vi "ReadConstantSpreadsheet.vi"(2 "error in":errorcluster, 3 "Constant":string="Drive Left Center", 4 "2020ConstantSpreadSheet":string[][](array[string])=[["Robot ID", "Motor ID", "Can Bus ID", "PWM Channel", "PDP Channel ID", "Breaker Needed", "Max. Allowed Current", "Solenoid Channel", "Analog Channel", "Digital I/O", "Notes", ""], ["981-2020", "Drive Right A", "11", "-1", "2", "40", "40", "-1", "-1", "-1", "", ""], ["981-2020", "Drive Right B", "12", "-1", "3", "40", "40", "-1", "-1", "-1", "", ""], ["981-2020", "Drive Left A", "13", "-1", "12", "40", "40", "-1", "-1", "-1", "", ""], ["981-2020", "Drive Left B", "14", "-1", "13", "40", "40", "-1", "-1", "-1", "", ""], ["981-2020", "Kicker", "15", "-1", "7", "20", "20", "-1", "-1", "-1", "", ""], ["981-2020", "Lift", "16", "-1", "6", "20", "20", "-1", "-1", "-1", "", ""], ["981-2020", "Shooter Left", "17", "-1", "1", "40", "40", "-1", "-1", "-1", "", ""], ["981-2020", "Shooter Right", "18", "-1", "0", "40", "40", "-1", "-1", "-1", "", ""], ["981-2020", "Pulley", "19", "-1", "5", "20", "20", "-1", "-1", "-1", "", ""], ["981-2020", "Intake", "20", "-1", "4", "20", "20", "-1", "-1", "-1", "", ""], ["981-2020", "Loader", "21", "-1", "11", "20", "20", "-1", "-1", "-1", "Changed name from spinner to the agreed name loader", ""], ["981-2020", "Winch", "22", "-1", "12", "20", "20", "-1", "-1", "-1", "", ""], ["981-2020", "Spare", "23", "-1", "8", "20", "20", "-1", "-1", "-1", "", ""], ["981S", "Drive Left Front", "0", "0", "0", "20", "20", "-1", "-1", "-1", "These are the IDs for the software sim of the 981 robot", ""], ["981S", "Drive Left Rear", "0", "1", "0", "20", "20", "-1", "-1", "-1", "", ""], ["981S", "Drive Right Front", "0", "0", "0", "20", "20", "-1", "-1", "-1", "", ""], ["981S", "Drive Right Rear", "0", "0", "0", "20", "20", "-1", "-1", "-1", "", ""], ["981S", "Gripper Left", "0", "0", "0", "20", "20", "-1", "-1", "-1", "", ""], ["981S", "Gripper Right", "0", "1", "0", "20", "20", "-1", "-1", "-1", "", ""], ["981S", "Winch Motor", "0", "0", "0", "20", "20", "-1", "-1", "-1", "", ""], ["981S", "Fork Lift Motor", "0", "1", "0", "20", "20", "-1", "-1", "-1", "", ""], ["981", "Drive Right A", "13", "-1", "13", "40", "28", "-1", "-1", "-1", "\"AKA", " drive right front\""], ["981", "Drive Right B", "14", "-1", "14", "40", "27", "-1", "-1", "-1", "\"AKA", " drive right rear\""], ["981", "Drive Left A", "11", "-1", "0", "40", "26", "-1", "-1", "-1", "\"AKA", " drive left front\""], ["981", "Drive Left B", "12", "-1", "1", "40", "25", "-1", "-1", "-1", "\"AKA", " drive left rear\""], ["981", "Winch", "15", "-1", "15", "40", "40", "-1", "-1", "-1", "", ""], ["981", "Arm", "17", "-1", "11", "30", "39", "-1", "-1", "-1", "", ""], ["981", "Arm Pot", "-1", "-1", "-1", "-1", "-1", "-1", "1", "-1", "Using Channel for Analog Input Channel", ""], ["981", "Arm Encoder", "-1", "-1", "-1", "-1", "-1", "-1", "-1", "0", "\"Digital IO for A", " add one for channel B\""], ["981", "Lights", "0", "0", "8", "20", "2", "-1", "-1", "-1", "\"20 amp is overkill", " but the minimum for the PDP\""], ["981", "Raspberry Pi", "0", "9", "10", "20", "3", "-1", "-1", "-1", "", ""], ["981", "Total PDP", "0", "0", "17", "120", "118", "-1", "-1", "-1", "", ""], ["981", "Extend Arm", "-1", "-1", "-1", "-1", "-1", "2", "-1", "-1", "", ""], ["981", "Retract Arm", "-1", "-1", "-1", "-1", "-1", "3", "-1", "-1", "", ""], ["981", "Shift Low", "-1", "-1", "-1", "-1", "-1", "6", "-1", "-1", "", ""], ["981", "Shift High", "-1", "-1", "-1", "-1", "-1", "7", "-1", "-1", "", ""], ["981", "Close Gripper", "-1", "-1", "-1", "-1", "-1", "0", "-1", "-1", "", ""], ["981", "Open Gripper", "-1", "-1", "-1", "-1", "-1", "1", "-1", "-1", "", ""], ["981", "Extend Hook", "-1", "-1", "-1", "-1", "-1", "4", "-1", "-1", "", ""], ["981", "Retract Hook", "-1", "-1", "-1", "-1", "-1", "5", "-1", "-1", "", ""], ["984", "Drive Left Front", "11", "-1", "0", "20", "20", "-1", "-1", "-1", "These are the IDS for the Rhino Robot practice robot", ""], ["984", "Drive Left Rear", "12", "-1", "1", "20", "20", "-1", "-1", "-1", "", ""], ["984", "Drive Left Center", "13", "-1", "2", "20", "20", "-1", "-1", "-1", "", ""], ["984", "Drive Right Front", "14", "-1", "12", "20", "20", "-1", "-1", "-1", "", ""], ["984", "Drive Right Rear", "15", "-1", "13", "20", "20", "-1", "-1", "-1", "", ""], ["984", "Drive Right Center", "16", "-1", "14", "20", "20", "-1", "-1", "-1", "", ""], ["984", "Gripper Left", "17", "-1", "8", "20", "20", "-1", "-1", "-1", "", ""], ["984", "Gripper Right", "18", "-1", "9", "20", "20", "-1", "-1", "-1", "", ""], ["984", "Winch", "19", "-1", "4", "20", "20", "-1", "-1", "-1", "", ""], ["984", "Fork Lift Motor", "20", "-1", "5", "20", "20", "-1", "-1", "-1", "", ""], ["985", "Drive Left Front", "11", "-1", "0", "20", "20", "-1", "-1", "-1", "These are the IDs for the AM drive practice robot", ""], ["985", "Drive Left Rear", "12", "-1", "1", "20", "20", "-1", "-1", "-1", "", ""], ["985", "Drive Right Front", "13", "-1", "2", "20", "20", "-1", "-1", "-1", "", ""], ["985", "Drive Right Rear", "14", "-1", "3", "20", "20", "-1", "-1", "-1", "", ""], ["985", "Gripper Left", "15", "-1", "10", "20", "20", "-1", "-1", "-1", "", ""], ["985", "Gripper Right", "16", "-1", "11", "20", "20", "-1", "-1", "-1", "", ""], ["985", "Winch Motor", "17", "-1", "14", "20", "20", "-1", "-1", "-1", "", ""], ["985", "Fork Lift Motor", "18", "-1", "5", "20", "20", "-1", "-1", "-1", "", ""], ["985SW", "Drive Right", "1", "-1", "1", "40", "20", "-1", "-1", "-1", "985 Summer Wheeled Robot right drive motor", ""], ["985SW", "Drive Left", "2", "-1", "1", "40", "20", "-1", "-1", "-1", "985 Summer Wheeled Robot left drive motor", ""], ["985SW", "Lift", "3", "-1", "1", "40", "20", "-1", "-1", "-1", "985 Lift Motor", ""]], 5 "Robot ID":string="984") -> (0 "error out":errorcluster, 1 "Constant Value":dbl)   [LabVIEW 2020]
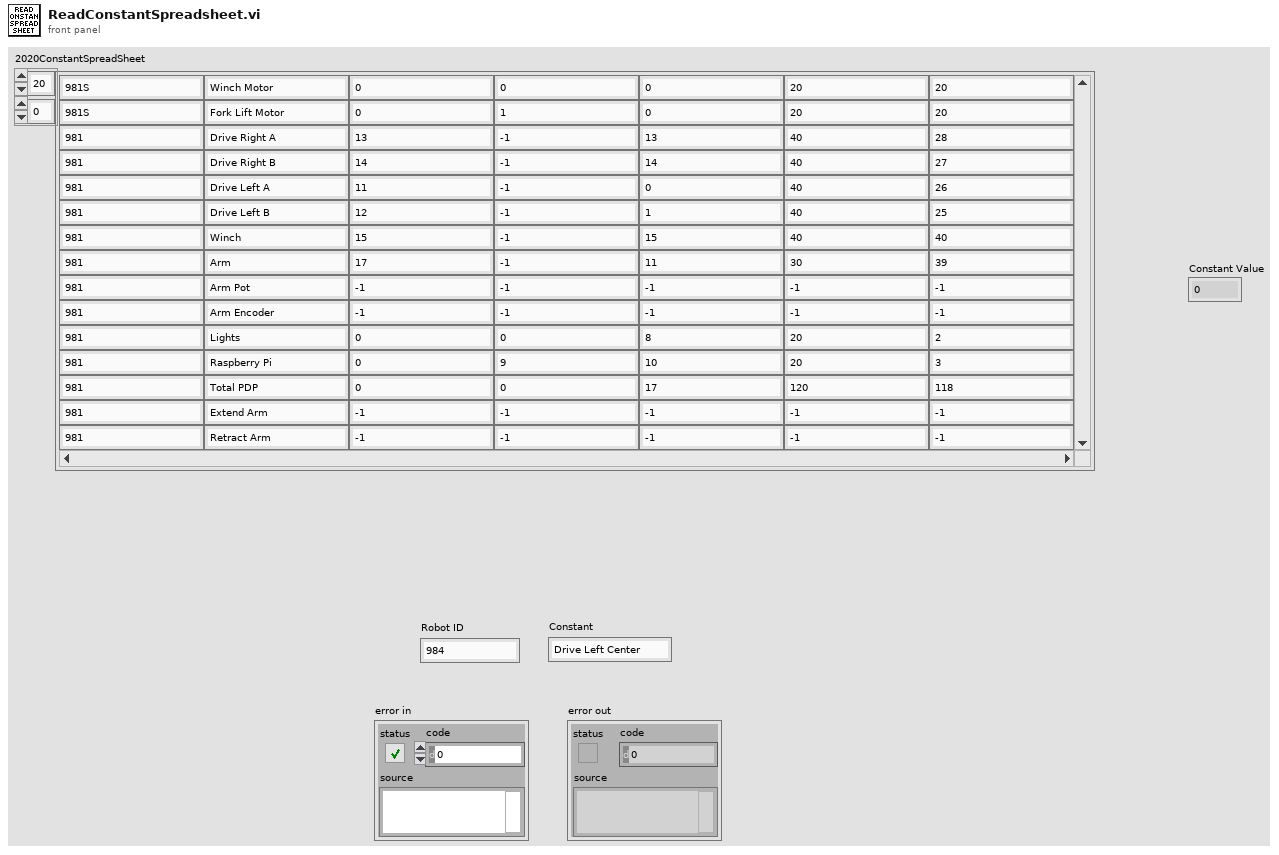
[diagram p1: front panel]
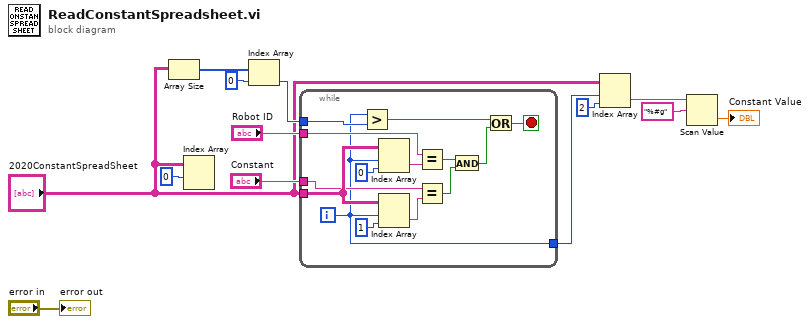
[diagram p0: block diagram]
diagram:
  n1 = Array Size(array="2020ConstantSpreadSheet") -> (size(s)=w12:i32[])
  n2 = Index Array(array="2020ConstantSpreadSheet", index (row)=0) -> ()  [unwired: 1 in, 1 out]
  n3 = Index Array(array=w12, index=0) -> (element=w10:i32)
  n4 = while {
    tunnel: "2020ConstantSpreadSheet" -> [w20]
    tunnel: w10 -> [w25]
    tunnel: "Robot ID" -> [w22]
    tunnel: "Constant" -> [w18]
    tunnel: [w14] -> w5
    i -> [w14]
    stop <- w24 stop-if-true
    n5 = Greater?(x=w14, y=w25) -> (0:w26:bool)
    n6 = Index Array(array=w20, index (row)=w14, index (col)=0 ("disabled index (col)")) -> (element=w23:string)
    n7 = Index Array(array=w20, index (row)=w14, index (col)=1) -> (element=w19:string)
    n8 = Equal?(x=w22, y=w23) -> (x = y?=w17:bool)
    n9 = Equal?(x=w18, y=w19) -> (x = y?=w16:bool)
    n10 = And(x=w17, y=w16) -> (x .and. y?=w15:bool)
    n11 = Or(x=w26, y=w15) -> (x .or. y?=w24:bool)
  }
  n12 = Index Array(array="2020ConstantSpreadSheet", index (row)=w5, index (col)=2 ("disabled index (col)")) -> (element=w2:string)
  n13 = Scan Value(string=w2, format string="%#g") -> (value=→"Constant Value":dbl)  [unwired: 1 in, 1 out]
  "error out" <- "error in"
